vi "Execute.vi"(8 "error in":errorcluster, 11 "Set O3 Level in":refnum<class "Set O3 Level.lvclass">) -> (0 "error out":errorcluster, 1 "Next Step?":bool, 2 "MSG":string, 3 "Set O3 Level out":refnum<class "Set O3 Level.lvclass">)   [LabVIEW 2015, in "Set O3 Level.lvclass"]
uses:
  Set O3 Level.lvclass
  Set O3 Level.lvclass/Set O3 Level.ctl
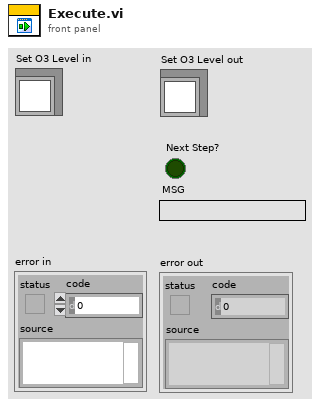
[diagram p1: front panel]
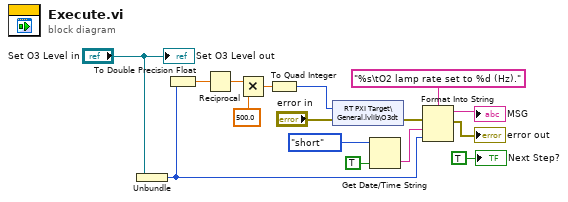
[diagram p0: block diagram]
diagram:
  n1 = Unbundle("Set O3 Level in") -> (w2:i32)
  n2 = To Double Precision Float(number=w2) -> (double precision float=w1:dbl)
  n3 = Reciprocal(x=w1) -> (1/x=w6:dbl)
  n4 = Multiply(x=w6, y=500.0) -> (x*y=w4:dbl)
  n5 = To Quad Integer(1:w4) -> (0:w3:i64)
  n6 = shared-variable "RT PXI Target\\General.lvlib\\O3dt"(w3, error in="error in") -> (error out=w9:errorcluster)
  n7 = Get Date/Time String(date format (0)=enum16{"short", "long", "abbreviated"}."short", want seconds? (F)=TRUE) -> (time string=w13:string)  [unwired: 1 in, 1 out]
  n8 = Format Into String(format string="%s\tO2 lamp rate set to %d (Hz).", error in=w9, w13, w2) -> (resulting string=→"MSG":string, error out=→"error out":errorcluster)  [unwired: 1 in]
  "Set O3 Level out" <- "Set O3 Level in"
  "Next Step?" <- TRUE ("Next Step?")
